vi "Read structureRef.vi"(8 "error in (no error)":errorcluster, 11 "Structure In":refnum<class "Structure.lvclass">) -> (0 "error out":errorcluster, 2 "nodeRef":refnum<vi>, 3 "Structure Out":refnum<class "Structure.lvclass">)   [LabVIEW 2023, in "TLC_Scripto.lvlib" / "Structure.lvclass"]
uses:
  Structure.lvclass
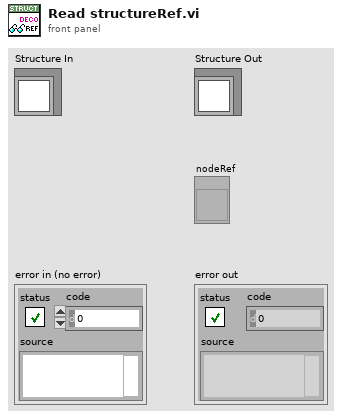
[diagram p1: front panel]
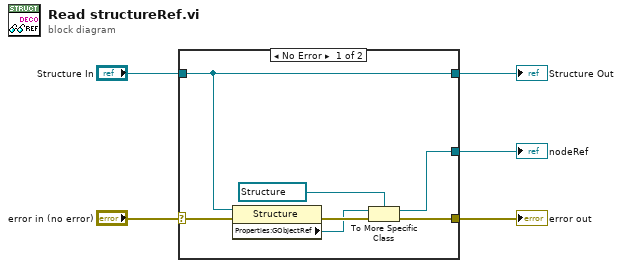
[diagram p0: block diagram]
diagram:
  n1 = case shown="No Error" "error in (no error)" {
    selector: "error in (no error)" -> [w8 w14]
    tunnel: [w7 w14] -> w4
    tunnel: [w9 w13] -> w2
    tunnel: "Structure In" -> [w9 w13]
    tunnel: [w6 _] -> w1
    frame No Error {
      n2 = property class="Structure"(reference=w9, error in=w8) -> (error out=w12:errorcluster, "Properties:GObjectRef"=w11:refnum<vi>)  [unwired: 1 out]
      n3 = To More Specific Class(target class=refnum<vi> refnum ("type"), reference=w11, error in=w12) -> (specific class reference=w6:refnum<vi>, error out=w7:errorcluster)
    }
    frame Error {
    }
  }
  "error out" <- w4
  "Structure Out" <- w2
  "nodeRef" <- w1
